vi "OAT Build Digital Tacho Info.vi"(0 "tacho counts":u32[](array[numeric]), 1 "synchronization type":u16(ring) items=["by sharing sample clock", "by using reference clock"], 2 "reset? (F)":bool, 5 "sample rate":dbl, 7 "counter task type":enum16{"period measurement", "event counting"}(ring)=enum."event counting", 9 "counter digit (32)":i32=32, 11 "error in (no error)":errorcluster, 12 "device info":T1 {"device type" items=["Custom"=0, "4472"=1, "4474"=11, "4461"=2, "4462"=12, "4464"=13, "449x"=7, "9232"=8, "9233"=3, "9234"=4, "9229"=5, "9239"=6]}, 13 "counter timebase [Hz]":dbl=20000000.0 format="%.0p") -> (4 "digital tacho info":T2={"tacho counts"=[], "counter timebase [Hz]"=1000.0, "counter task type"=enum."event counting", "counter digit (32)"=32}, 15 "error out":errorcluster)   [LabVIEW 2017, in "SoundVib_TachProcess.lvlib"]
doc: "Builds a digital tachometer signal information cluster that compensates for the input filter delay in the sound or vibration acquisition channel. You can use the output of this VI as an input for the OAT Digital Tacho Process VI."
uses:
  <vilib>/addons/Sound and Vibration/Order Analysis/Tach Process/SoundVib_TachProcess.lvlib
  <vilib>/addons/Sound and Vibration/Order Analysis/Tach Process/SubVIs/digital tach info.ctl
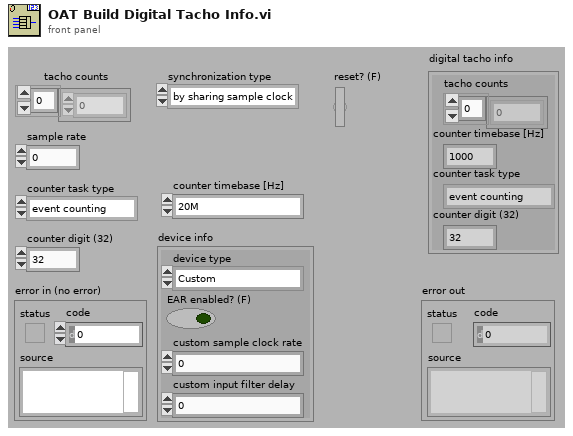
[diagram p1: front panel]
types:
  T1 = cluster{"device type":u16, "EAR enabled? (F)":bool, "custom sample clock rate":dbl, "custom input filter delay":dbl}
  T2 = typedef "SoundVib_TachProcess.lvlib/digital tach info.ctl" = cluster{"tacho counts":i64[], "counter timebase [Hz]":dbl, "counter task type":enum16{"period measurement", "event counting"}, "counter digit (32)":i32}
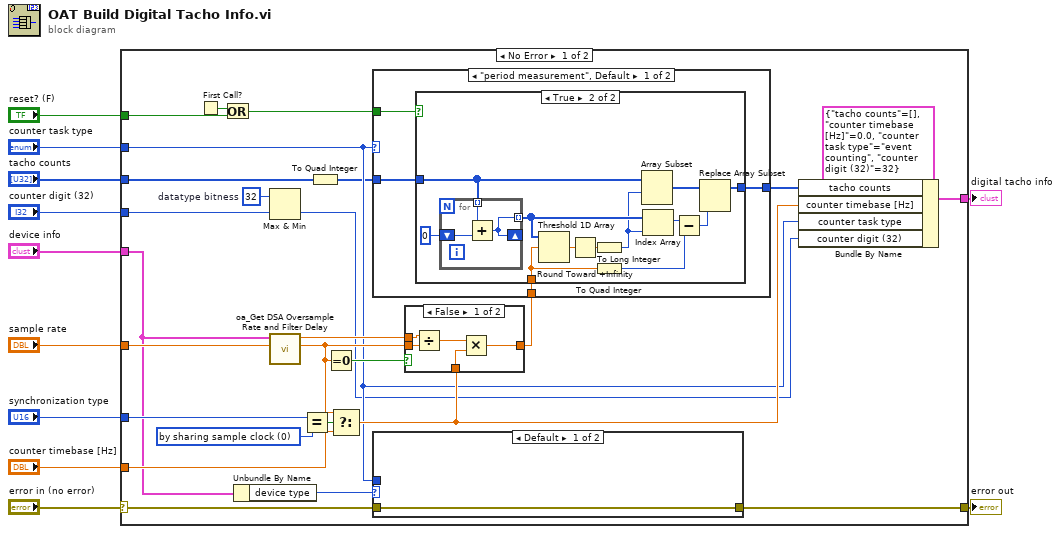
[diagram p0: block diagram]
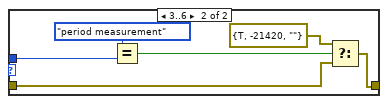
[diagram p2: hidden frame]
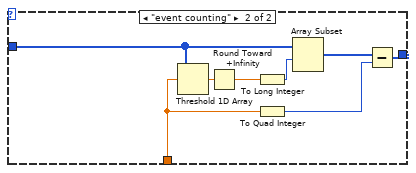
[diagram p5: hidden frame]
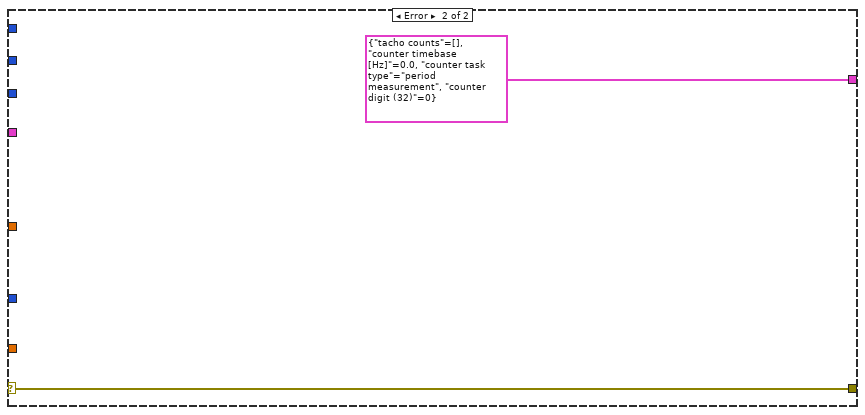
[diagram p6: hidden frame]
diagram:
  n1 = case shown="No Error" "error in (no error)" {
    selector: "error in (no error)" -> [w20 w80]
    tunnel: [w18 w80] -> w10
    tunnel: "sample rate" -> [w23 _]
    tunnel: "counter task type" -> [w19 _]
    tunnel: "tacho counts" -> [w16 _]
    tunnel: "counter digit (32)" -> [w14 _]
    tunnel: [w36 T2 {"tacho counts"=[], "counter timebase [Hz]"=0.0, "counter task type"=enum."period measurement", "counter digit (32)"=0} ("digital tacho info")] -> w5
    tunnel: "reset? (F)" -> [w33 _]
    tunnel: "synchronization type" -> [w32 _]
    tunnel: "counter timebase [Hz]" -> [w29 _]
    tunnel: "device info" -> [w22 _]
    frame No Error {
      w13 = 32  # datatype bitness
      w31 = u16 0 items=["by sharing sample clock", "by using reference clock"] ("synchronization type")
      n2 = First Call?() -> (First Call?: T/F=w35:bool)
      n3 = Or(x=w35, y=w33) -> (x .or. y?=w34:bool)
      n4 = Unbundle By Name(w22) -> ("device type"=w21:u16)
      n5 = Max & Min(x=w13, y=w14) -> (min(x,y)=w12:i32)  [unwired: 1 out]
      n6 = call <vilib>:"oa_Get DSA Oversample Rate and Filter Delay.vi"("sample rate"=w23, "device info"=w22) -> ("SampClkTimebase"=w25:dbl, "input delay"=w24:dbl)  [unwired: 8 in]
      n7 = Equal?(x=w32, y=w31) -> (x = y?=w30:bool)
      n8 = To Quad Integer(1:w16) -> (0:w15:i64[])
      n9 = Equal To 0?(x=w25) -> (x = 0?=w26:bool)
      n10 = Select(t=w25, s=w30, f=w29) -> (s? t:f=w28:dbl)
      n11 = case shown="Default" w21 {
        tunnel: w20 -> [w38 w41]
        tunnel: w19 -> [_ w43]
        tunnel: [w38 w40] -> w18
        frame Default {
        }
        frame 3..6 {
          n12 = Equal?(x=enum16{"period measurement", "event counting"}."period measurement" ("y"), y=w43) -> (x = y?=w42:bool)
          n13 = Select(t=errorcluster {"status"=TRUE, "code"=-21420, "source"=""}, s=w42, f=w41) -> (s? t:f=w40:errorcluster)
        }
      }
      n14 = case shown="False" w26 {
        tunnel: w24 -> [w49 _]
        tunnel: w28 -> [w47 _]
        tunnel: w25 -> [w46 w50]
        tunnel: [w45 w50] -> w27
        frame False {
          n15 = Divide(x=w49, y=w46) -> (x/y=w48:dbl)
          n16 = Multiply(x=w48, y=w47) -> (x*y=w45:dbl)
        }
        frame True {
        }
      }
      n17 = case shown="\"period measurement\", Default" w19 {
        tunnel: w15 -> [w51 w76]
        tunnel: [w53 w75] -> w37
        tunnel: w27 -> [w54 w71]
        tunnel: w34 -> [w52 _]
        frame "period measurement", Default {
          n18 = case shown="True" w52 {
            tunnel: w54 -> [_ w58]
            tunnel: w51 -> [w55 w56]
            tunnel: [w55 w60] -> w53
            frame False {
            }
            frame True {
              n19 = for {
                shift-right: [w69] -> _
                shift-left: i64 0 -> [w70]
                tunnel: [w69] -> w67 mode=indexing
                tunnel: w56 -> [w68] mode=indexing
                n20 = Add(x=w68, y=w70) -> (x+y=w69:i64)
              }
              n21 = Threshold 1D Array(2:w58, 3:w67) -> (0:w66:dbl)  [unwired: 1 in]
              n22 = Round Toward +Infinity(x=w66) -> (ceil(x): smallest int >= x=w64:dbl)
              n23 = To Long Integer(number=w64) -> (32bit integer=w57:i32)
              n24 = To Quad Integer(1:w58) -> (0:w59:i64)
              n25 = Array Subset(array=w56, index=w57) -> (w62:i64[])  [unwired: 1 in]
              n26 = Index Array(array=w67, index=w57) -> (element=w63:i64)
              n27 = Subtract(x=w63, y=w59) -> (x-y=w61:i64)
              n28 = Replace Array Subset(array=w62, new element=w61) -> (w60:i64[])  [unwired: 1 in]
            }
          }
        }
        frame "event counting" {
          n29 = Threshold 1D Array(2:w71, 3:w76) -> (0:w78:dbl)  [unwired: 1 in]
          n30 = Round Toward +Infinity(x=w78) -> (ceil(x): smallest int >= x=w77:dbl)
          n31 = To Long Integer(number=w77) -> (32bit integer=w73:i32)
          n32 = To Quad Integer(1:w71) -> (0:w74:i64)
          n33 = Array Subset(array=w76, index=w73) -> (w72:i64[])  [unwired: 1 in]
          n34 = Subtract(x=w72, y=w74) -> (x-y=w75:i64[])
        }
      }
      n35 = Bundle By Name(cluster=T2 {"tacho counts"=[], "counter timebase [Hz]"=0.0, "counter task type"=enum."event counting", "counter digit (32)"=32} ("digital tacho info"), "tacho counts"=w37, "counter timebase [Hz]"=w28, "counter task type"=w19, "counter digit (32)"=w12) -> (w36:T2)
    }
    frame Error {
    }
  }
  "digital tacho info" <- w5
  "error out" <- w10
